vi "SortidaAnalogicaUSB.vi"(0 "VelocitatAssaig":refnum<vi>, 5 "stop":refnum<vi>, 11 "VelMaxima":refnum<vi>) -> ()   [LabVIEW 2017]
uses:
  <vilib>/DAQmx/write.llb/DAQmx Write (Analog DBL 1Chan 1Samp).vi
  <vilib>/DAQmx/miscellaneous.llb/DAQmx Fill In Error Info.vi
  <resource>/objmgr/daqmx.rc
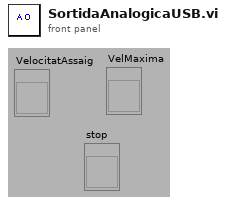
[diagram p1: front panel]
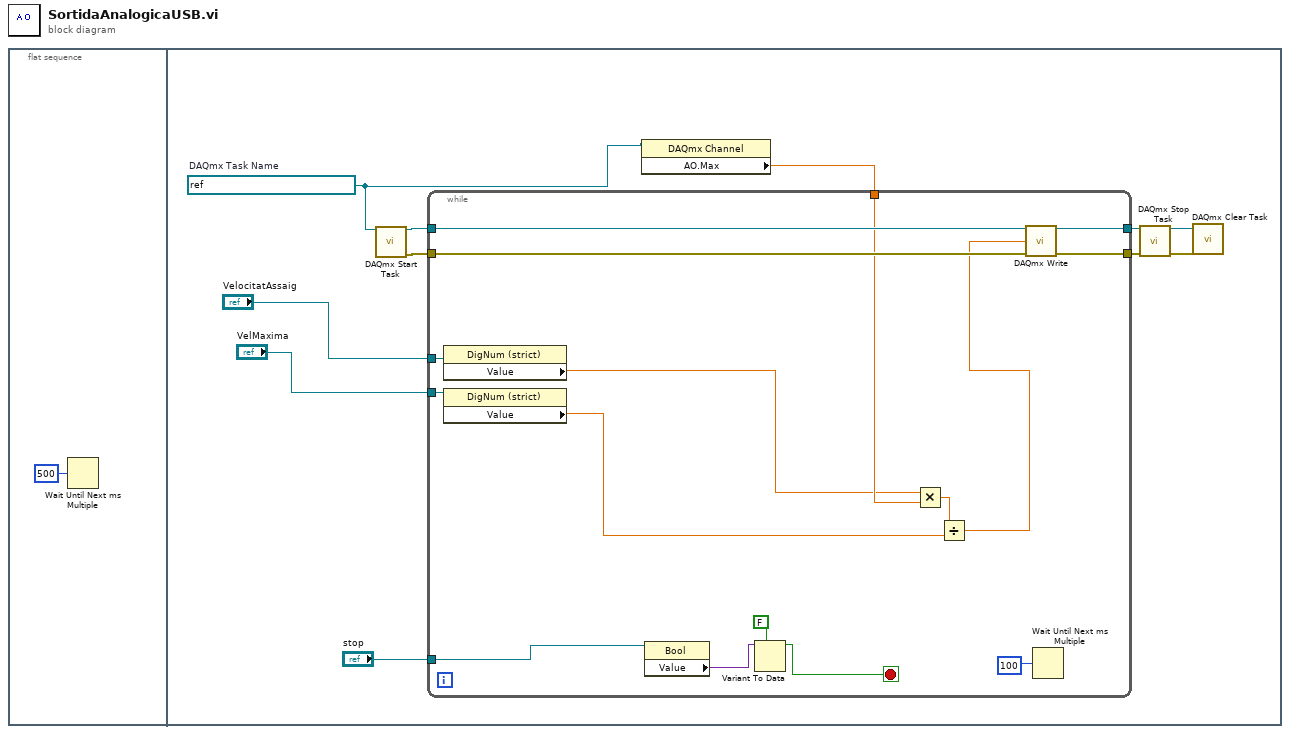
[diagram p0: block diagram]
diagram:
  n1 = flat-sequence {
    frame #0 {
      n2 = Wait Until Next ms Multiple(millisecond multiple=u32 500) -> ()  [unwired: 1 out]
    }
    frame #1 {
      w5 = refnum<k21> "TallGuants_USBAnalogOut"  # DAQmx Task Name
      n3 = call <vilib>:"DAQmx Start Task.vi"("task/channels in"=w5) -> ("task out"=w12:refnum<k21>, "error out"=w10:errorcluster)  [unwired: 13 in]
      n4 = property class="DAQmx Channel"(reference=w5) -> ("AO.Max"=w4:dbl)  [unwired: 1 in, 2 out]
      n5 = while {
        tunnel: w12 -> [w20]
        tunnel: [w19] -> w11
        tunnel: w10 -> [w22]
        tunnel: [w28] -> w9
        tunnel: "stop" -> [w26]
        tunnel: "VelocitatAssaig" -> [w21]
        tunnel: "VelMaxima" -> [w17]
        tunnel: w4 -> [w16]
        stop <- w23 stop-if-true
        n6 = property class="DigNum (strict)"(reference=w21) -> ("Value"=w15:sgl)  [unwired: 1 in, 2 out]
        n7 = property class="DigNum (strict)"(reference=w17) -> ("Value"=w14:sgl)  [unwired: 1 in, 2 out]
        n8 = property class="Bool"(reference=w26) -> ("Value"=w25:variant)  [unwired: 1 in, 2 out]
        n9 = Variant To Data(type=FALSE ("stop"), Variant=w25) -> (data=w23:bool)  [unwired: 1 in, 1 out]
        n10 = Multiply(x=w15, y=w16) -> (x*y=w13:dbl)
        n11 = Divide(x=w13, y=w14) -> (x/y=w18:dbl)
        n12 = call-poly <vilib>:"DAQmx Write.vi"("task/channels in"=w20, "data"=w18, "error in"=w22) -> ("task out"=w19:refnum<k21>, "error out"=w28:errorcluster)  [unwired: 10 in, 1 out]
        n13 = Wait Until Next ms Multiple(millisecond multiple=u32 100) -> ()  [unwired: 1 out]
      }
      n14 = call <vilib>:"DAQmx Stop Task.vi"("task/channels in"=w11, "error in"=w9) -> ("task out"=w3:refnum<k21>, "error out"=w2:errorcluster)  [unwired: 12 in]
      n15 = call <vilib>:"DAQmx Clear Task.vi"("task in"=w3, "error in"=w2) -> ()  [unwired: 13 in, 1 out]
    }
  }
